vi "Read OOB RX.vi"(8 "error in (no error)":errorcluster, 11 "CIFCorePlugin in":refnum<class "CIFCorePlugin.lvclass">) -> (0 "error out":errorcluster, 3 "CIFCorePlugin out":refnum<class "CIFCorePlugin.lvclass">)   [LabVIEW 2021, in "CIFCorePlugin.lvclass"]
uses:
  CIFCorePlugin.lvclass
  CIFCorePlugin.lvclass/CIFCorePlugin.ctl
  CIFUtilities/CIFOutOfBand/CIFOutOfBand.lvclass/CIFOutOfBand.ctl
  Typedef/Energized States.ctl
  CIFUtilities/CIFOutOfBand/Read OOB DVR.vi
  CIFCoreOOB/OOB_Rx/Private/Command Settings.vi
  CIFCoreOOB/OOB_Rx/Private/Read Payload.vi
  CIFUtilities/CIFOutOfBand/Accessors/Read Local OOB Data.vi
  CIFCoreOOB/OOB_Rx/CIFCoreOOB_Rx.lvclass
  D:/dev/CIF-LVCore/src/CIFUtilities/CIFOutOfBand/CIFOutOfBand.lvclass
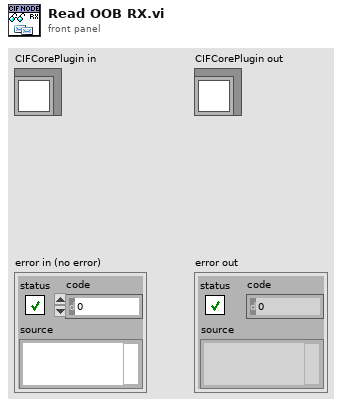
[diagram p1: front panel]
types:
  T1 = typedef "CIFCorePlugin.lvclass/Energized States.ctl" = enum16{"Listen", "Prepare", "Execute", "Housekeep", "Cleanup", "Destroy"}
  T2 = typedef "CIFCoreOOB_Rx.lvclass/OOB Core Commands.ctl" = enum8{"Start", "StartFTE", "Pause", "Stop", "RefreshStats", "UpdateConfig"}
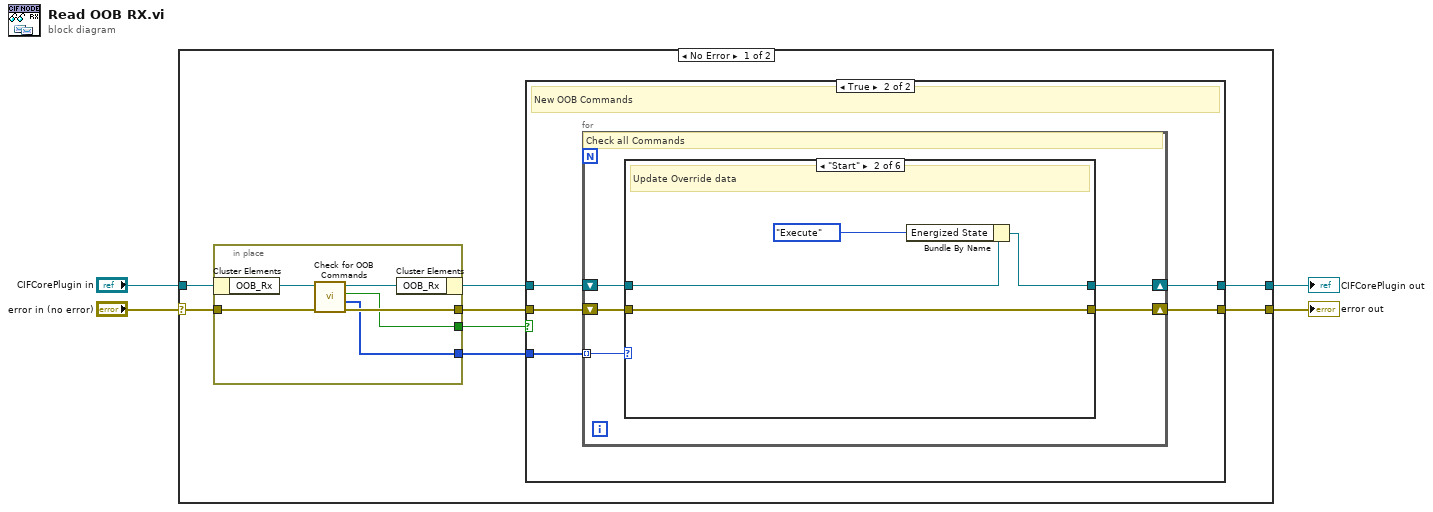
[diagram p0: block diagram]
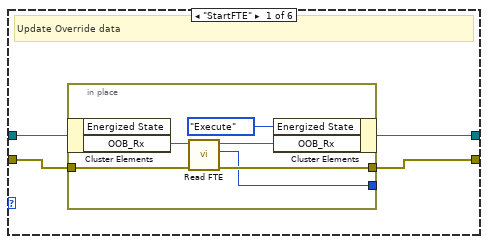
[diagram p3: hidden frame]
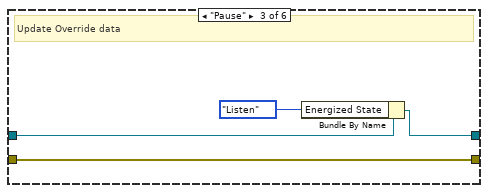
[diagram p4: hidden frame]
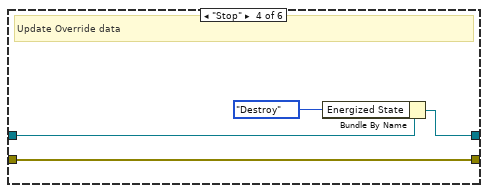
[diagram p5: hidden frame]
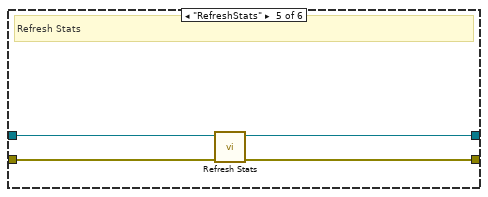
[diagram p6: hidden frame]
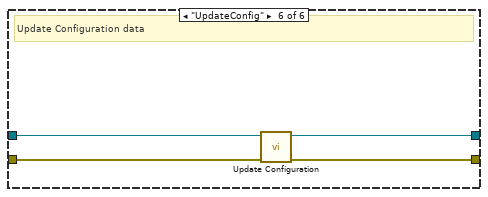
[diagram p7: hidden frame]
diagram:
  n1 = case shown="No Error" "error in (no error)" {
    selector: "error in (no error)" -> [w11 w62]
    tunnel: [w5 w62] -> w3
    tunnel: [w7 w61] -> w1
    tunnel: "CIFCorePlugin in" -> [w12 w61]
    frame No Error {
      n2 = in-place {
        in-place-border: w11 -> [w59]
        in-place-border: [w57] -> w6
        in-place-border: [w56] -> w9
        in-place-border: [w55] -> w10
        n3 = in-place-cluster #1(w12) -> ("OOB_Rx"=w60:refnum<class "CIFCoreOOB_Rx.lvclass">)
        n4 = call "Check for OOB Commands.vi"("error in (no error)"=w59, "CoreOOB_Rx in"=w60) -> ("error out"=w57:errorcluster, "Commands"=w56:T2[], "New Commands"=w55:bool, "CoreOOB_Rx out"=w58:refnum<class "CIFCoreOOB_Rx.lvclass">)  [unwired: 6 in]
        n5 = in-place-cluster #1("OOB_Rx"=w58) -> (w8:refnum<class "CIFCorePlugin.lvclass">)
      }
      n6 = case shown="True" w10 {
        tunnel: w9 -> [_ w19]
        tunnel: w8 -> [w14 w18]
        tunnel: [w14 w16] -> w7
        tunnel: w6 -> [w13 w17]
        tunnel: [w13 w15] -> w5
        frame False {
          # "No new OOB Commands"
        }
        frame True {
          # "New OOB Commands"
          n7 = for {
            tunnel: w19 -> [w24] mode=indexing
            shift-right: [w21] -> w16
            shift-left: w18 -> [w22]
            shift-right: [w20] -> w15
            shift-left: w17 -> [w23]
            # "Check all Commands"
            n8 = case shown="\"Start\"" w24 {
              tunnel: w23 -> [w27 w35 w42 w46 w49 w53]
              tunnel: w22 -> [w28 w36 w41 w45 w50 w54]
              tunnel: [w26 w38 w40 w44 w48 w52] -> w21
              tunnel: [w25 w35 w42 w46 w47 w51] -> w20
              frame "StartFTE" {
                # "Update Override data"
                n9 = in-place {
                  in-place-border: w27 -> [w32]
                  in-place-border: [w31] -> w25
                  in-place-border: [w29] -> _
                  n10 = in-place-cluster #2(w28) -> ("OOB_Rx"=w34:refnum<class "CIFCoreOOB_Rx.lvclass">)  [unwired: 1 out]
                  n11 = call "Read FTE.vi"("error in"=w32, "CoreOOB_Rx in"=w34) -> ("error out"=w31:errorcluster, "FTE"=w29:u64, "CoreOOB_Rx out"=w33:refnum<class "CIFCoreOOB_Rx.lvclass">)  [unwired: 7 in]
                  n12 = in-place-cluster #2("Energized State"=Energized_States."Execute" ("Energized States in"), "OOB_Rx"=w33) -> (w26:refnum<class "CIFCorePlugin.lvclass">)
                }
              }
              frame "Start" {
                # "Update Override data"
                n13 = Bundle By Name(cluster=w36, "Energized State"=Energized_States."Execute" ("Energized States in")) -> (w38:refnum<class "CIFCorePlugin.lvclass">)
              }
              frame "Pause" {
                # "Update Override data"
                n14 = Bundle By Name(cluster=w41, "Energized State"=Energized_States."Listen" ("Energized States in")) -> (w40:refnum<class "CIFCorePlugin.lvclass">)
              }
              frame "Stop" {
                # "Update Override data"
                n15 = Bundle By Name(cluster=w45, "Energized State"=Energized_States."Destroy" ("Energized States in")) -> (w44:refnum<class "CIFCorePlugin.lvclass">)
              }
              frame "RefreshStats" {
                # "Refresh Stats"
                n16 = call "Refresh Stats.vi"("error in (no error)"=w49, "CIFCorePlugin in"=w50) -> ("error out"=w47:errorcluster, "CIFCorePlugin out"=w48:refnum<class "CIFCorePlugin.lvclass">)  [unwired: 8 in]
              }
              frame "UpdateConfig" {
                # "Update Configuration data"
                n17 = call-dynamic "Update Configuration.vi"("error in (no error)"=w53, "CIFTemplateNode in"=w54) -> ("error out"=w51:errorcluster, "CIFTemplateNode out"=w52:refnum<class "CIFCorePlugin.lvclass">)  [unwired: 8 in]
              }
            }
          }
        }
      }
    }
    frame Error {
    }
  }
  "error out" <- w3
  "CIFCorePlugin out" <- w1
